vi "pos2centerRadi.vi"(9 "pos fin":dbl, 11 "pos init":dbl) -> (1 "semi diff (r)":dbl, 3 "semi sum (C)":dbl)   [LabVIEW 2023]
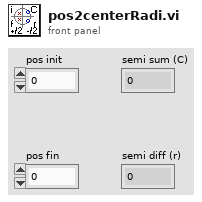
[diagram p1: front panel]
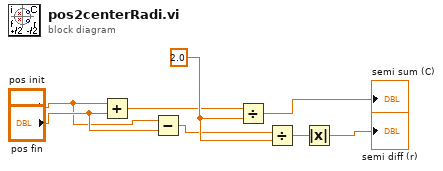
[diagram p0: block diagram]
diagram:
  w6 = 2.0 ("y")
  n1 = Add(x="pos init", y="pos fin") -> (x+y=w1:dbl)
  n2 = Subtract(x="pos init", y="pos fin") -> (x-y=w5:dbl)
  n3 = Divide(x=w1, y=w6) -> (x/y=→"semi sum (C)":dbl)
  n4 = Divide(x=w5, y=w6) -> (x/y=w7:dbl)
  n5 = Absolute Value(x=w7) -> (abs(x)=→"semi diff (r)":dbl)
